vi "Initialize.vi"(7 "deviceIdentifier":string, 8 "error in (no error)":errorcluster, 9 "top file path":path, 10 "shw file path":path, 11 "topologyName":string) -> (0 "error out":errorcluster, 3 "Route Manager out":refnum<class "slscsl.lvclass">)   [LabVIEW 2015, in "slscsl.lvclass"]
uses:
  slscsl.lvclass
  slscsl.lvclass/slscsl.ctl
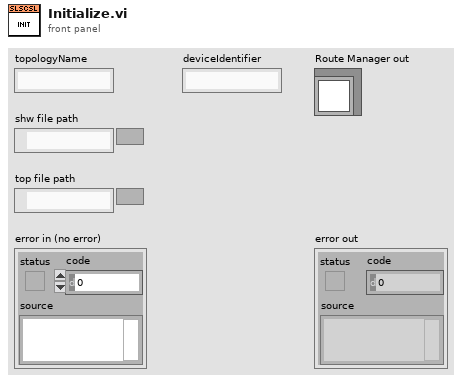
[diagram p1: front panel]
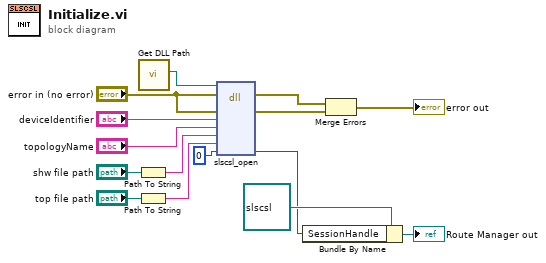
[diagram p0: block diagram]
diagram:
  n1 = Path To String(path="shw file path") -> (string=w3:string)
  n2 = Path To String(path="top file path") -> (string=w4:string)
  n3 = call "Get DLL Path.vi"() -> ("slscsl DLL Path"=w2:path)  [unwired: 11 in]
  n4 = dll-call lib="?" fn="slscsl_open"(path in=w2, error in="error in (no error)", "errorCluster"="error in (no error)", "deviceIdentifier"="deviceIdentifier", "topologyName"="topologyName", "shwFilePath"=w3, "topFilePath"=w4, "sessionHandlePtr"=u64 0) -> (error out=w6:errorcluster, "errorCluster"=w5:errorcluster, "sessionHandlePtr"=w1:u64)  [unwired: 6 in, 1 out]
  n5 = Bundle By Name(cluster=refnum<class "slscsl.lvclass"> refnum ("Route Manager out"), "SessionHandle"=w1) -> (→"Route Manager out":refnum<class "slscsl.lvclass">)
  n6 = Merge Errors(w6, w5) -> (→"error out":errorcluster)
